vi "PAN_RunRespSet.vi"(6 "nodeID":string, 7 "cmd in":string, 8 "error in (no error)":errorcluster, 10 "resp in":string, 11 "type specifier VI Refnum (for type only)":refnum<vi>) -> (0 "error out":errorcluster, 2 "resp out":string, 3 "type specifier VI Refnum out":refnum<vi>)   [LabVIEW 2016]
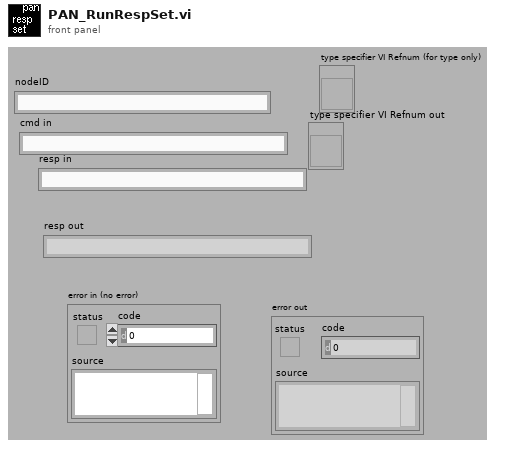
[diagram p1: front panel]
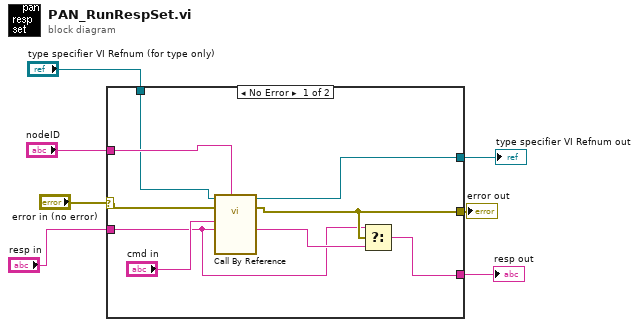
[diagram p0: block diagram]
diagram:
  n1 = case shown="No Error" "error in (no error)" {
    selector: "error in (no error)" -> [w16 w19]
    tunnel: [w11 w19] -> w7
    tunnel: "resp in" -> [w8 w18]
    tunnel: [w9 w18] -> w5
    tunnel: "nodeID" -> [w14 _]
    tunnel: "type specifier VI Refnum (for type only)" -> [w13 w17]
    tunnel: [w12 w17] -> w1
    frame No Error {
      n2 = call-by-ref "?"(reference=w13, error in=w16, "nodeID"=w14, "resp in"=w8, "cmd in"="cmd in") -> (reference out=w12:refnum<vi>, error out=w11:errorcluster, "resp out"=w10:string)  [unwired: 8 in]
      n3 = Select(t=w8, s=w11, f=w10) -> (s? t:f=w9:string)
    }
    frame Error {
    }
  }
  "error out" <- w7
  "resp out" <- w5
  "type specifier VI Refnum out" <- w1
